vi "新秒至时间处理.vi"(10 "数值":dbl) -> (2 "连接的字符串":string)   [LabVIEW 2016]
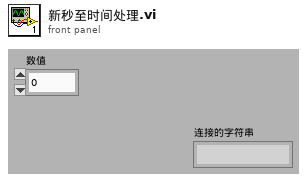
[diagram p1: front panel]
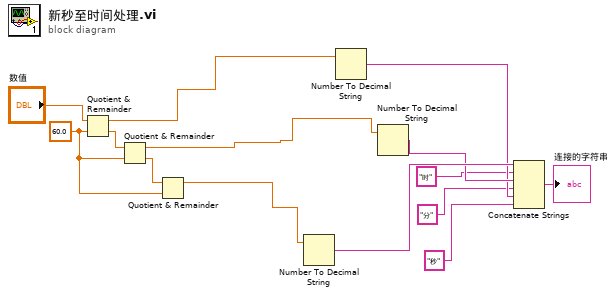
[diagram p0: block diagram]
diagram:
  w11 = 60.0 ("y")
  n1 = Quotient & Remainder(x="数值", y=w11) -> (x-y*floor(x/y)=w8:dbl, floor(x/y)=w13:dbl)
  n2 = Quotient & Remainder(x=w13, y=w11) -> (x-y*floor(x/y)=w9:dbl, floor(x/y)=w12:dbl)
  n3 = Quotient & Remainder(x=w12, y=w11) -> (x-y*floor(x/y)=w10:dbl)  [unwired: 1 out]
  n4 = Number To Decimal String(number=w10) -> (decimal integer string=w7:string)  [unwired: 1 in]
  n5 = Number To Decimal String(number=w8) -> (decimal integer string=w4:string)  [unwired: 1 in]
  n6 = Number To Decimal String(number=w9) -> (decimal integer string=w6:string)  [unwired: 1 in]
  n7 = Concatenate Strings(w7, "时", w6, "分", w4, "秒") -> (→"连接的字符串":string)
